vi "ObtainRequestEvents.vi"(8 "Error":errorcluster[](array[cluster])) -> (0 "Error":errorcluster[](array[cluster]), 3 "clRequestEvents":T1)   [LabVIEW 2014, in "Visualization.lvlib" / "VisualizeBase_class.lvclass"]
uses:
  VisualizeBase_class.lvclass
  clRequestEvents.ctl
  clUserEventType.ctl
panel:
  # "If you want to add other Request Events, open this typedef, copy an existing event and rename it to your event name."
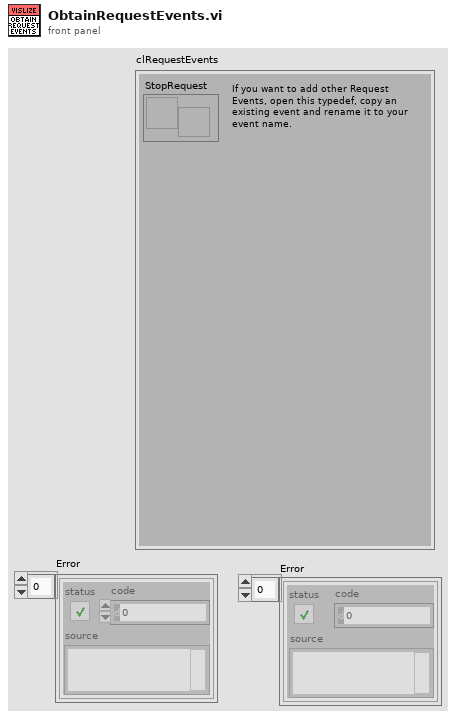
[diagram p1: front panel]
types:
  T1 = typedef "Visualization.lvlib/VisualizeBase_class.lvclass/clRequestEvents.ctl" = cluster{"StopRequest":refnum<user-event>}
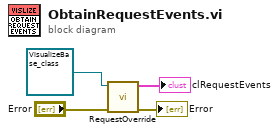
[diagram p0: block diagram]
diagram:
  n1 = call-dynamic "RequestOverride.vi"("Error in"="Error", "Visualize"=refnum<class "VisualizeBase_class.lvclass"> refnum ("Visualization.lvlib:VisualizeBase_class.lvclass")) -> ("Error out"=→"Error":errorcluster[], "RequestEvents"=→"clRequestEvents":T1)  [unwired: 8 in]
